vi "Laboratory_VI1.vi"() -> ()   [LabVIEW 2022 SP3]
panel:
  out "Thermometer (deg F)":dbl(slide) scale=0.0..100.0
  in  "Thermometer (deg C)":dbl(slide) scale=0.0..100.0
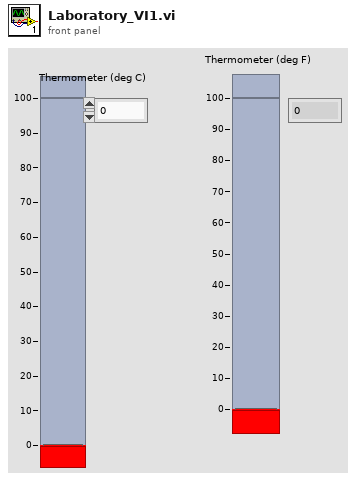
[diagram p1: front panel]
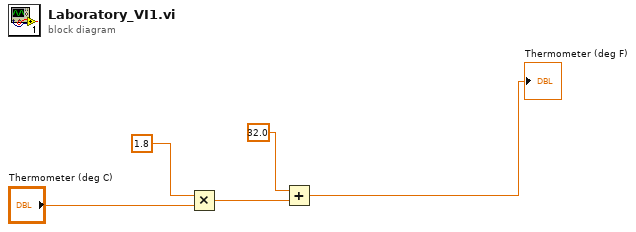
[diagram p0: block diagram]
diagram:
  n1 = Multiply(x=1.8, y="Thermometer (deg C)") -> (x*y=w2:dbl)
  n2 = Add(x=32.0, y=w2) -> (x+y=→"Thermometer (deg F)":dbl)
